vi "tag to string.vi"(8 "error in":errorcluster, 11 "tag descriptor in":refnum<class "tag descriptor.lvclass">) -> (0 "error out":errorcluster, 2 "tag string":string, 3 "tag descriptor out":refnum<class "tag descriptor.lvclass">)   [LabVIEW 2013, in "tag bus.lvlib" / "tag descriptor.lvclass"]
uses:
  tag descriptor.lvclass
  tag descriptor.lvclass/tag descriptor.ctl
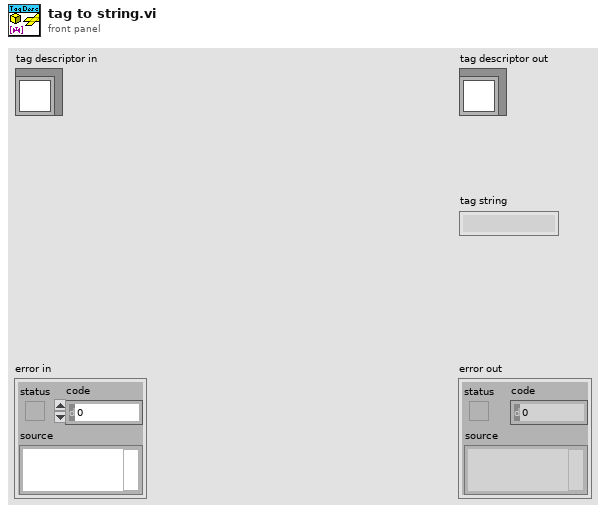
[diagram p1: front panel]
types:
  T1 = typedef "tag bus.lvlib/tag descriptor.lvclass/Data Type.ctl" = enum16{"Double", "Single", "I64", "I32", "I16", "I8", "U64", "U32", "U16", "U8", "Boolean", "String", "Array of Double", "Array of Single", "Array of I64", "Array of I32", "Array of I16", "Array of I8", "Array of U64", "Array of U32", "Array of U16", "Array of U8", "Array of Boolean", "Array of String"}
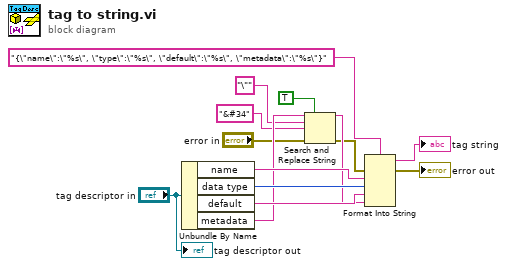
[diagram p0: block diagram]
diagram:
  n1 = Unbundle By Name("tag descriptor in") -> ("name"=w10:string, "data type"=w11:T1, "default"=w12:string, "metadata"=w7:string)
  n2 = Search and Replace String(replace all?=TRUE ("replace all? (F)"), input string=w7, search string="\"", replace string="&#34" ("replace string (\"\")"), error in="error in") -> (result string=w3:string, error out=w1:errorcluster)  [unwired: 3 in, 2 out]
  n3 = Format Into String(format string="{\"name\":\"%s\", \"type\":\"%s\", \"default\":\"%s\", \"metadata\":\"%s\"}", error in=w1, w10, w11, w12, w3) -> (resulting string=→"tag string":string, error out=→"error out":errorcluster)  [unwired: 1 in]
  "tag descriptor out" <- "tag descriptor in"
